vi "concatenar_cadenas_clase.vi"() -> ()   [LabVIEW 2020]
panel:
  in  "Cadena De Entrada":string="CH0:2; CH1:12; CH2:170."
  out "Entrada 3":dbl
  out "after substring 3":string
  out "after substring 2":string
  out "Entrada 2":dbl
  out "Entrada 1":dbl
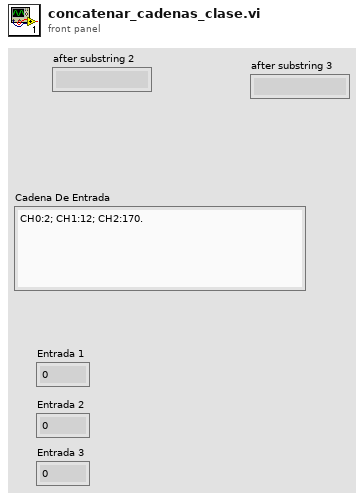
[diagram p1: front panel]
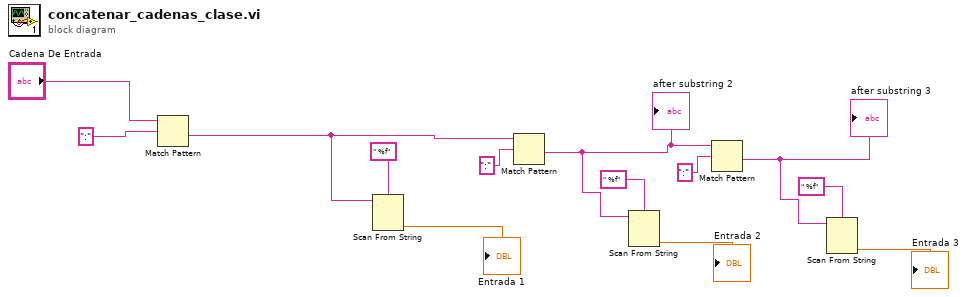
[diagram p0: block diagram]
diagram:
  n1 = Match Pattern(string="Cadena De Entrada", regular expression=":") -> (after substring=w9:string)  [unwired: 1 in, 3 out]
  n2 = Scan From String "Scan From String"(format string=" %f", input string=w9) -> (output 1=→"Entrada 1":dbl)  [unwired: 3 in, 3 out]
  n3 = Match Pattern(string=w9, regular expression=":") -> (after substring=w1:string)  [unwired: 1 in, 3 out]
  "after substring 2" <- w1
  n4 = Scan From String "Scan From String"(format string=" %f", input string=w1) -> (output 1=→"Entrada 2":dbl)  [unwired: 3 in, 3 out]
  n5 = Match Pattern(string=w1, regular expression=":") -> (after substring=w5:string)  [unwired: 1 in, 3 out]
  "after substring 3" <- w5
  n6 = Scan From String "Scan From String"(format string=" %f", input string=w5) -> (output 1=→"Entrada 3":dbl)  [unwired: 3 in, 3 out]
